vi "Result.vi"(8 "error in (no error)":errorcluster, 10 "Result":T1={"Name"="", "Description"="", "Status"=enum."Passed", "Result Type"=enum."Test Suite", "Execution Time"=0.0, "Data"={"Expected"=variant, "Actual"=variant, "Delta"=variant}}, 11 "Execution API In":refnum<class "Execution API.lvclass">) -> (0 "error out":errorcluster)   [LabVIEW 2020, in "Execution API.lvclass"]
uses:
  Execution API.lvclass
  Core/Result/Result.ctl
  Core/Result/Status.ctl
  Core/Result/Type.ctl
  Execution API.lvclass/Execution API.ctl
  Plugin/Plugin.lvclass
  Core/Result/Result.lvlib
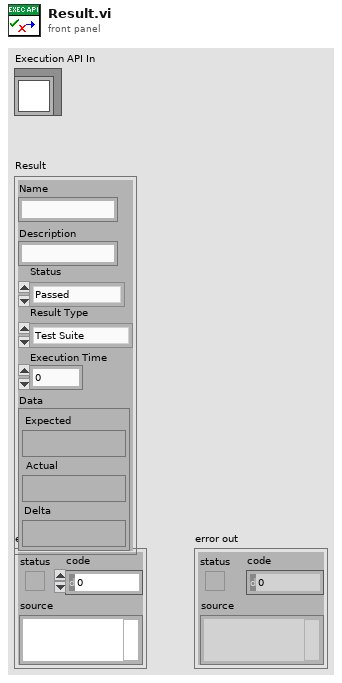
[diagram p1: front panel]
types:
  T1 = typedef "Result.lvlib/Result.ctl" = cluster{"Name":string, "Description":string, "Status":T2, "Result Type":T3, "Execution Time":dbl, "Data":cluster{"Expected":variant, "Actual":variant, "Delta":variant}}
  T2 = typedef "Result.lvlib/Status.ctl" = enum16{"", "Passed", "Failed", "Error", "Skipped", "Setup Error", "Broken", "Teardown Error"}
  T3 = typedef "Result.lvlib/Type.ctl" = enum16{"Test Case", "Test Suite", "Test Run", "Pass", "Fail", "Skip", "Pass if", "Fail if", "Pass if Error", "Fail if Error", "Pass if Equal", "Fail if Equal"}
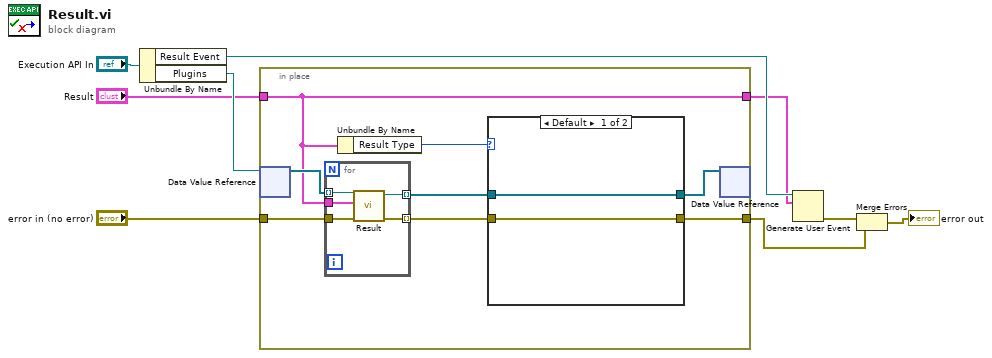
[diagram p0: block diagram]
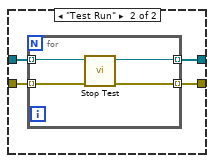
[diagram p2: hidden frame]
diagram:
  n1 = Unbundle By Name("Execution API In") -> ("Result Event"=w8:refnum<user-event>, "Plugins"=w5:refnum<data-value>)
  n2 = in-place {
    in-place-border: "error in (no error)" -> [w11]
    in-place-border: "Result" -> [w10]
    in-place-border: [w12] -> w3
    in-place-border: [w10] -> w1
    n3 = in-place-dvr #1(w5) -> (w16:refnum<class "Plugin.lvclass">[])  [unwired: 1 out]
    n4 = for {
      tunnel: w10 -> [w22]
      tunnel: w16 -> [w21] mode=indexing
      tunnel: [w20] -> w15 mode=indexing
      tunnel: [w19] -> w13 mode=indexing
      tunnel: w11 -> [w18]
      n5 = call-dynamic "Result.vi"("error in (no error)"=w18, "Result"=w22, "Plugin In"=w21) -> ("error out"=w19:errorcluster, "Plugin Out"=w20:refnum<class "Plugin.lvclass">)  [unwired: 7 in]
    }
    n6 = Unbundle By Name(w10) -> ("Result Type"=w17:T3)
    n7 = case shown="Default" w17 {
      tunnel: w15 -> [w24 w28]
      tunnel: [w24 w27] -> w14
      tunnel: w13 -> [w23 w26]
      tunnel: [w23 w25] -> w12
      frame Default {
      }
      frame "Test Run" {
        n8 = for {
          tunnel: w28 -> [w32] mode=indexing
          tunnel: [w31] -> w27 mode=indexing
          tunnel: w26 -> [w30] mode=indexing
          tunnel: [w29] -> w25 mode=indexing
          n9 = call-dynamic "Stop Test.vi"("error in (no error)"=w30, "Plugin in"=w32) -> ("error out"=w29:errorcluster, "Plugin out"=w31:refnum<class "Plugin.lvclass">)  [unwired: 8 in]
        }
      }
    }
    n10 = in-place-dvr #1(w14) -> ()  [unwired: 2 out]
  }
  n11 = Generate User Event(user event=w8, event data cluster=w1) -> (error out=w7:errorcluster)  [unwired: 2 in, 1 out]
  n12 = Merge Errors(w7, w3) -> (→"error out":errorcluster)
